vi "Method_Const.vi"(4 "String":string, 5 "Value A":refnum<class "Abs_String.lvclass">) -> (1 "Result":refnum<class "Abs_Boolean.lvclass">)   [LabVIEW 2021, in "Not Equal_STR.lvclass"]
uses:
  Not Equal_STR.lvclass
  Abs_Types/String/Abs_String.lvclass
  Abs_Types/Boolean/Abs_Boolean.lvclass
  C:/TSA/LV_Abstract/Source/Functions/Support/Compare/Two Term/STR/AbsComp_Two Term_STR.lvclass
  C:/Program Files (x86)/National Instruments/LabVIEW 2021/vi.lib/TSA/Abstract Data Classes/Abs_Types/Boolean/Abs_Boolean.lvclass
  Support/Compare/Two Term/STR/AbsComp_Two Term_STR.lvclass/AbsComp_Two Term_STR.ctl
  Support/Compare/Two Term/STR/Properties/Write String A.vi
  Support/Compare/Two Term/STR/Properties/Write String B.vi
  Constants/Support/Str/Const_Str.lvclass
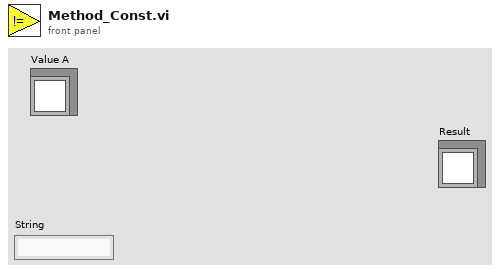
[diagram p1: front panel]
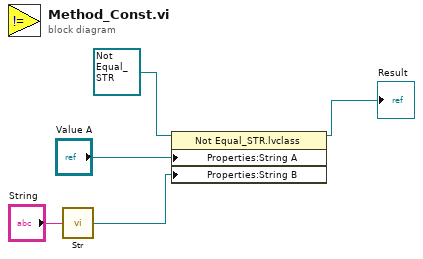
[diagram p0: block diagram]
diagram:
  n1 = call "Str.vi"("String"="String") -> ("Abs_String.lvclass"=w2:refnum<class "Abs_String.lvclass">)  [unwired: 4 in]
  n2 = property class="Not Equal_STR.lvclass"(reference=refnum<class "Not Equal_STR.lvclass"> refnum ("Greater 0_U64.lvclass"), "Properties:String A"="Value A", "Properties:String B"=w2) -> (reference out=→"Result":refnum<class "Not Equal_STR.lvclass">)  [unwired: 1 in, 1 out]
